vi "sub_NMEA_msg_parser.vi"(9 "VTG String ($이후~\\n이전)":string, 10 "RMC String ($이후~\\n이전)":string, 11 "GGA String ($이후~\\n이전)":string) -> (1 "VTG cluster":T3, 2 "RMC cluster":T2, 3 "GGA cluster":T1)   [LabVIEW 2020]
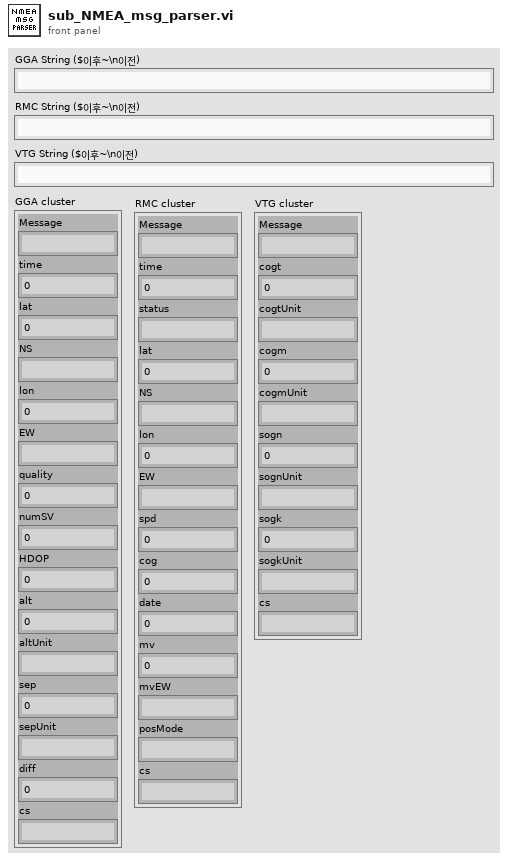
[diagram p1: front panel]
types:
  T1 = cluster{"Message":string, "time":dbl, "lat":dbl, "NS":string, "lon":dbl, "EW":string, "quality":u8, "numSV":u8, "HDOP":dbl, "alt":dbl, "altUnit":string, "sep":dbl, "sepUnit":string, "diff":i32, "cs":string}
  T2 = cluster{"Message":string, "time":dbl, "status":string, "lat":dbl, "NS":string, "lon":dbl, "EW":string, "spd":dbl, "cog":dbl, "date":u32, "mv":dbl, "mvEW":string, "posMode":string, "cs":string}
  T3 = cluster{"Message":string, "cogt":dbl, "cogtUnit":string, "cogm":dbl, "cogmUnit":string, "sogn":dbl, "sognUnit":string, "sogk":dbl, "sogkUnit":string, "cs":string}
  T4 = cluster{"string array[0]":string, "string array[1]":string, "string array[2]":string, "string array[3]":string, "string array[4]":string, "string array[5]":string, "string array[6]":string, "string array[7]":string, "string array[8]":string, "string array[9]":string, "string array[10]":string, "string array[11]":string, "string array[12]":string, "string array[13]":string, "string array[14]":string}
  T5 = cluster{"string array[0]":string, "string array[1]":string, "string array[2]":string, "string array[3]":string, "string array[4]":string, "string array[5]":string, "string array[6]":string, "string array[7]":string, "string array[8]":string, "string array[9]":string, "string array[10]":string, "string array[11]":string, "string array[12]":string, "string array[13]":string}
  T6 = cluster{"string array[0]":string, "string array[1]":string, "string array[2]":string, "string array[3]":string, "string array[4]":string, "string array[5]":string, "string array[6]":string, "string array[7]":string, "string array[8]":string, "string array[9]":string}
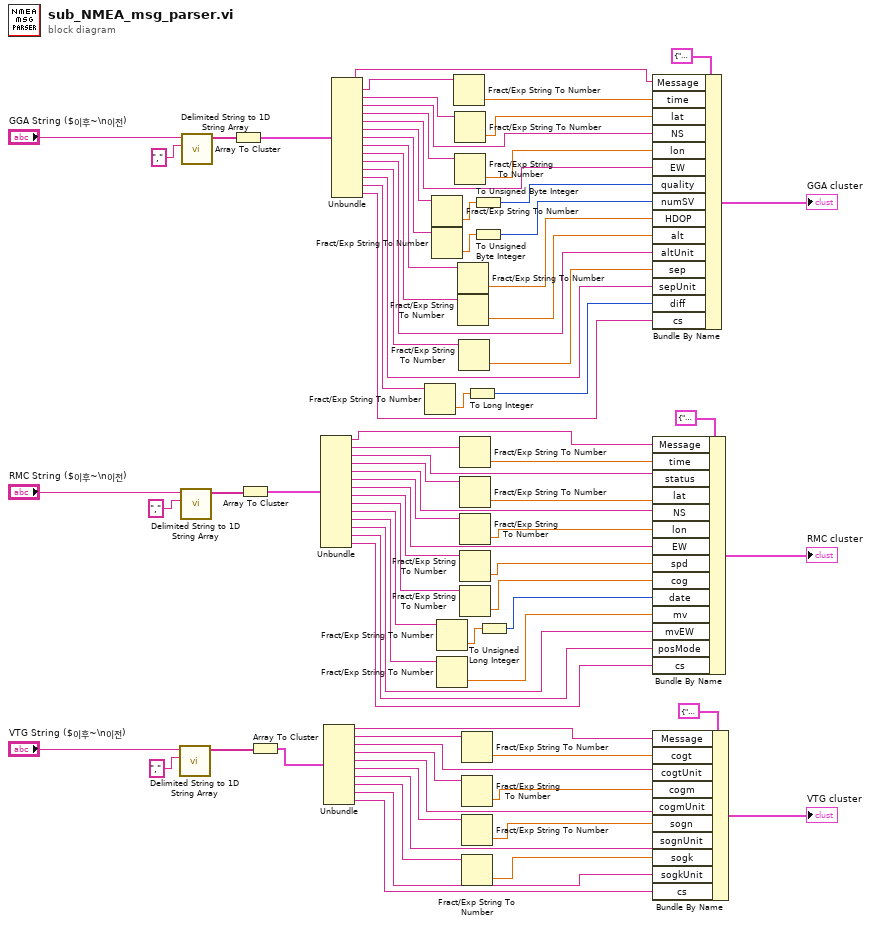
[diagram p0: block diagram]
diagram:
  n1 = call <vilib>:"Delimited String to 1D String Array.vi"("delimiter"=",", "delimited string"="VTG String ($이후~\\n이전)") -> ("string array"=w29:string[])  [unwired: 9 in]
  n2 = call <vilib>:"Delimited String to 1D String Array.vi"("delimiter"=",", "delimited string"="RMC String ($이후~\\n이전)") -> ("string array"=w24:string[])  [unwired: 9 in]
  n3 = call <vilib>:"Delimited String to 1D String Array.vi"("delimiter"=",", "delimited string"="GGA String ($이후~\\n이전)") -> ("string array"=w2:string[])  [unwired: 9 in]
  n4 = Array To Cluster(array=w2) -> (cluster=w3:T4)
  n5 = Array To Cluster(array=w24) -> (cluster=w49:T5)
  n6 = Array To Cluster(array=w29) -> (cluster=w64:T6)
  n7 = Unbundle(w49) -> ("string array[0]"=w63:string, "string array[1]"=w50:string, "string array[2]"=w51:string, "string array[3]"=w52:string, "string array[4]"=w53:string, "string array[5]"=w54:string, "string array[6]"=w55:string, "string array[7]"=w56:string, "string array[8]"=w57:string, "string array[9]"=w58:string, "string array[10]"=w59:string, "string array[11]"=w60:string, "string array[12]"=w61:string, "string array[13]"=w62:string)
  n8 = Unbundle(w64) -> ("string array[0]"=w74:string, "string array[1]"=w65:string, "string array[2]"=w66:string, "string array[3]"=w67:string, "string array[4]"=w68:string, "string array[5]"=w69:string, "string array[6]"=w70:string, "string array[7]"=w71:string, "string array[8]"=w72:string, "string array[9]"=w73:string)
  n9 = Unbundle(w3) -> ("string array[0]"=w48:string, "string array[1]"=w47:string, "string array[2]"=w46:string, "string array[3]"=w45:string, "string array[4]"=w44:string, "string array[5]"=w43:string, "string array[6]"=w42:string, "string array[7]"=w41:string, "string array[8]"=w40:string, "string array[9]"=w39:string, "string array[10]"=w38:string, "string array[11]"=w37:string, "string array[12]"=w36:string, "string array[13]"=w35:string, "string array[14]"=w34:string)
  n10 = Fract/Exp String To Number(string=w35) -> (number=w13:dbl)  [unwired: 3 in, 1 out]
  n11 = Fract/Exp String To Number(string=w42) -> (number=w6:dbl)  [unwired: 3 in, 1 out]
  n12 = Fract/Exp String To Number(string=w41) -> (number=w8:dbl)  [unwired: 3 in, 1 out]
  n13 = Fract/Exp String To Number(string=w58) -> (number=w21:dbl)  [unwired: 3 in, 1 out]
  n14 = Fract/Exp String To Number(string=w59) -> (number=w19:dbl)  [unwired: 3 in, 1 out]
  n15 = Fract/Exp String To Number(string=w47) -> (number=w4:dbl)  [unwired: 3 in, 1 out]
  n16 = Fract/Exp String To Number(string=w46) -> (number=w31:dbl)  [unwired: 3 in, 1 out]
  n17 = Fract/Exp String To Number(string=w44) -> (number=w32:dbl)  [unwired: 3 in, 1 out]
  n18 = Fract/Exp String To Number(string=w40) -> (number=w10:dbl)  [unwired: 3 in, 1 out]
  n19 = Fract/Exp String To Number(string=w39) -> (number=w11:dbl)  [unwired: 3 in, 1 out]
  n20 = Fract/Exp String To Number(string=w37) -> (number=w12:dbl)  [unwired: 3 in, 1 out]
  n21 = Fract/Exp String To Number(string=w50) -> (number=w17:dbl)  [unwired: 3 in, 1 out]
  n22 = Fract/Exp String To Number(string=w52) -> (number=w75:dbl)  [unwired: 3 in, 1 out]
  n23 = Fract/Exp String To Number(string=w54) -> (number=w33:dbl)  [unwired: 3 in, 1 out]
  n24 = Fract/Exp String To Number(string=w56) -> (number=w22:dbl)  [unwired: 3 in, 1 out]
  n25 = Fract/Exp String To Number(string=w57) -> (number=w18:dbl)  [unwired: 3 in, 1 out]
  n26 = Fract/Exp String To Number(string=w65) -> (number=w25:dbl)  [unwired: 3 in, 1 out]
  n27 = Fract/Exp String To Number(string=w67) -> (number=w26:dbl)  [unwired: 3 in, 1 out]
  n28 = Fract/Exp String To Number(string=w69) -> (number=w27:dbl)  [unwired: 3 in, 1 out]
  n29 = Fract/Exp String To Number(string=w71) -> (number=w28:dbl)  [unwired: 3 in, 1 out]
  n30 = To Long Integer(number=w13) -> (32bit integer=w14:i32)
  n31 = To Unsigned Byte Integer(number=w6) -> (unsigned 8bit integer=w7:u8)
  n32 = To Unsigned Byte Integer(number=w8) -> (unsigned 8bit integer=w9:u8)
  n33 = To Unsigned Long Integer(number=w21) -> (unsigned 32bit integer=w20:u32)
  n34 = Bundle By Name(cluster=T1 {"Message"="", "time"=0.0, "lat"=0.0, "NS"="", "lon"=0.0, "EW"="", "quality"=0, "numSV"=0, "HDOP"=0.0, "alt"=0.0, "altUnit"="", "sep"=0.0, "sepUnit"="", "diff"=0, "cs"=""}, "Message"=w48, "time"=w4, "lat"=w31, "NS"=w45, "lon"=w32, "EW"=w43, "quality"=w7, "numSV"=w9, "HDOP"=w10, "alt"=w11, "altUnit"=w38, "sep"=w12, "sepUnit"=w36, "diff"=w14, "cs"=w34) -> (→"GGA cluster":T1)
  n35 = Bundle By Name(cluster=T2 {"Message"="", "time"=0.0, "status"="", "lat"=0.0, "NS"="", "lon"=0.0, "EW"="", "spd"=0.0, "cog"=0.0, "date"=0, "mv"=0.0, "mvEW"="", "posMode"="", "cs"=""}, "Message"=w63, "time"=w17, "status"=w51, "lat"=w75, "NS"=w53, "lon"=w33, "EW"=w55, "spd"=w22, "cog"=w18, "date"=w20, "mv"=w19, "mvEW"=w60, "posMode"=w61, "cs"=w62) -> (→"RMC cluster":T2)
  n36 = Bundle By Name(cluster=T3 {"Message"="", "cogt"=0.0, "cogtUnit"="", "cogm"=0.0, "cogmUnit"="", "sogn"=0.0, "sognUnit"="", "sogk"=0.0, "sogkUnit"="", "cs"=""}, "Message"=w74, "cogt"=w25, "cogtUnit"=w66, "cogm"=w26, "cogmUnit"=w68, "sogn"=w27, "sognUnit"=w70, "sogk"=w28, "sogkUnit"=w72, "cs"=w73) -> (→"VTG cluster":T3)
